vi "AddNormalPulseVoltammetry.vi"(0 "deviceName":string, 1 "channel":u8, 2 "repeats":u16=1, 3 "quietTime":sgl, 4 "quietTimeSamplingInterval":sgl=1.0, 5 "startVoltage":sgl, 6 "isStartVoltageVsOCP":bool, 7 "error in (no error)":errorcluster, 8 "endVoltage":sgl, 9 "isEndVoltageVsOCP":bool, 10 "vStep":sgl, 11 "pulseWidth":sgl, 12 "pulsePeriod":sgl, 13 "approxMaxCurrent":sgl=inf, 14 "isAutoRange":bool=TRUE, 15 "alphaFactor":sgl=75.0) -> (27 "error out":errorcluster)   [LabVIEW 2018]
doc: "EXPORT void AisAddNormalPulseVoltammetry(const char* deviceName, uint8_t channel, uint16_t repeats, float quietTime, float quietTimeSamplingInterval, float startVoltage, bool isStartVoltageVsOCP, float endVoltage, bool isEndVoltageVsOCP, float vStep, float pulseWidth, float pulsePeriod, float approxMaxCurrent, bool isAutoRange, float alphaFactor);"
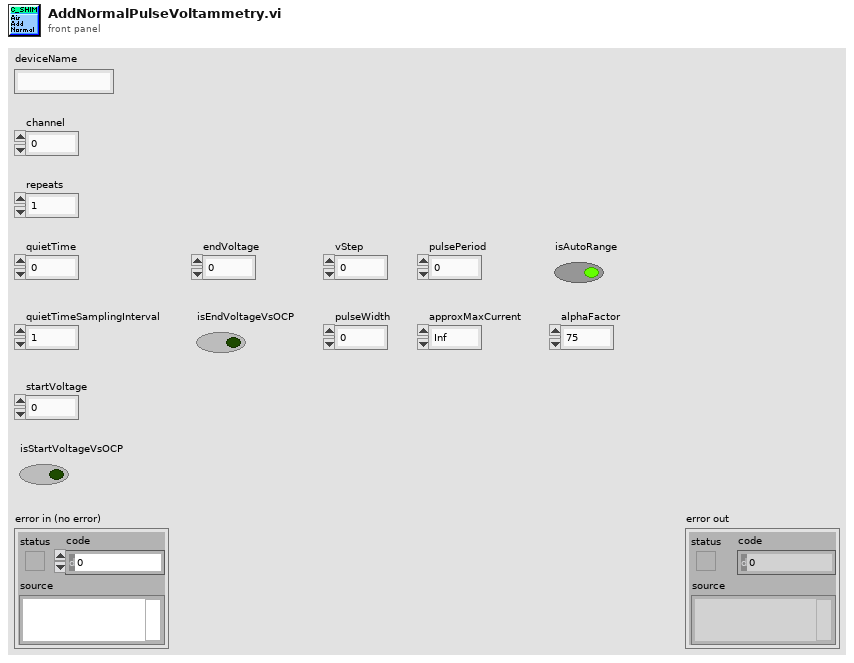
[diagram p1: front panel]
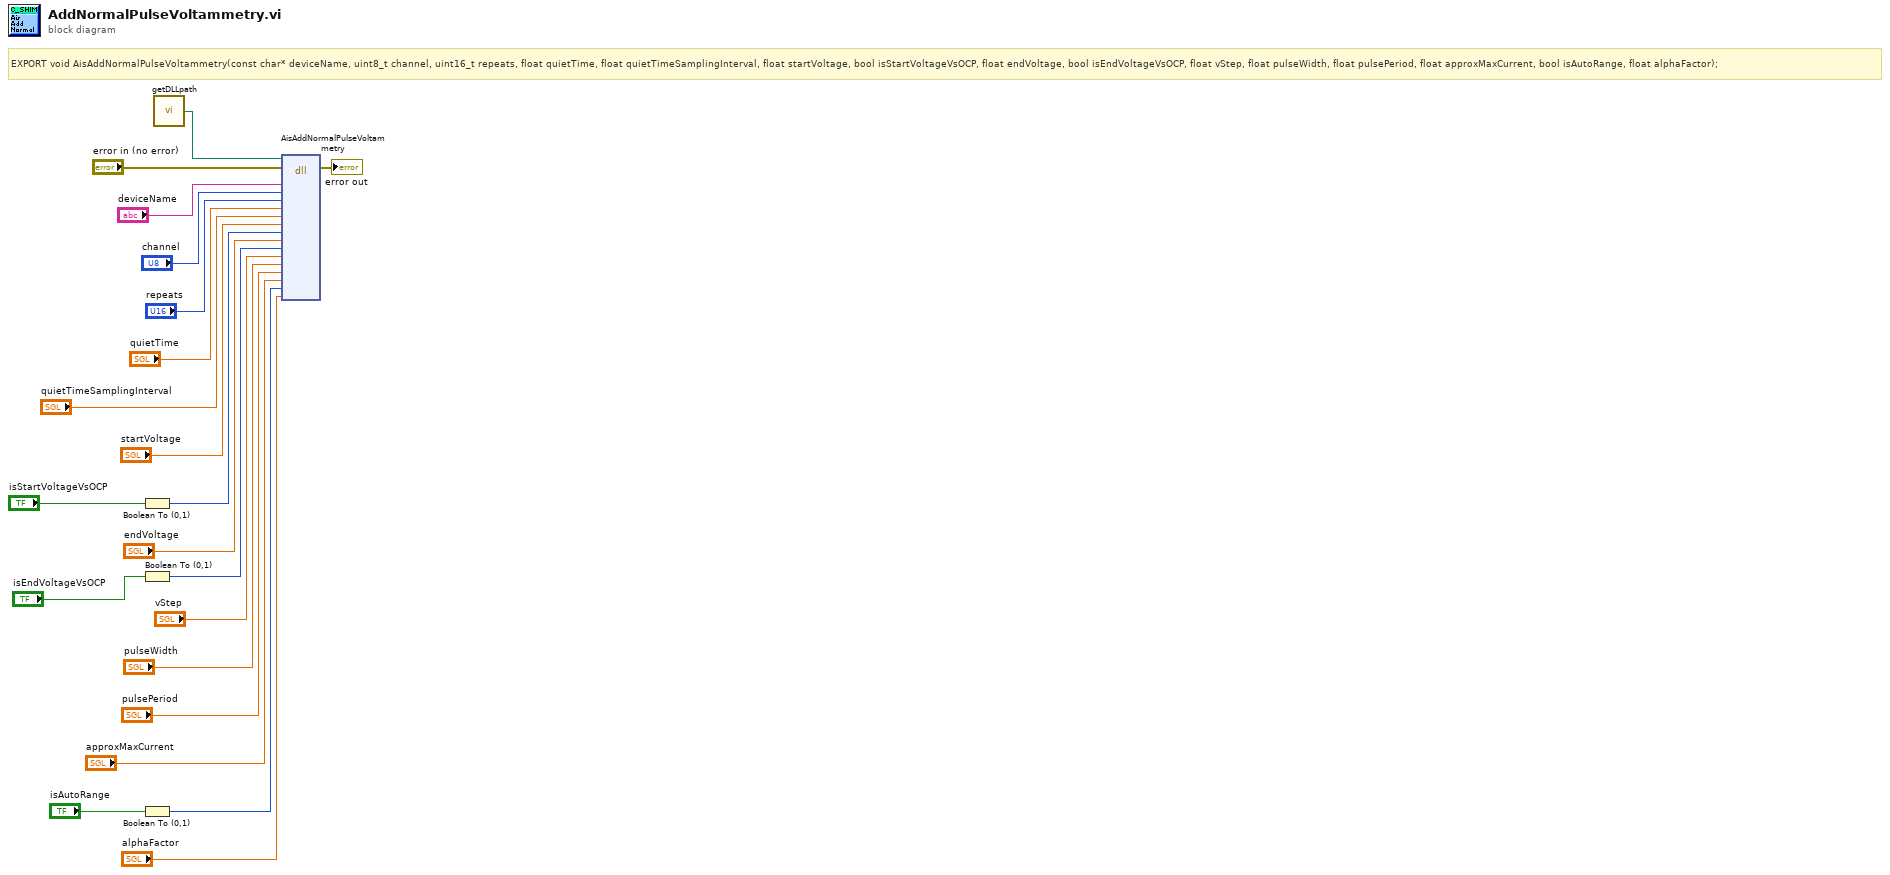
[diagram p0: block diagram]
diagram:
  # "EXPORT void AisAddNormalPulseVoltammetry(const char* deviceName, uint8_t channel, uint16_t repeats, float quietTime, float quietTimeSamplingInterval, float startVoltage, bool isStartVoltageVsOCP, float endVoltage, bool isEndVoltageVsOCP, float vStep, float pulseWidth, float pulsePeriod, float approxMaxCurrent, bool isAutoRange, float alphaFactor);"
  n1 = Boolean To (0,1)(Boolean="isStartVoltageVsOCP") -> (0, 1=w14:i16)
  n2 = Boolean To (0,1)(Boolean="isEndVoltageVsOCP") -> (0, 1=w11:i16)
  n3 = Boolean To (0,1)(Boolean="isAutoRange") -> (0, 1=w5:i16)
  n4 = call "getDLLpath.vi"() -> ("DLL_Path"=w1:path)
  n5 = dll-call lib="?" fn="AisAddNormalPulseVoltammetry"(path in=w1, error in="error in (no error)", "deviceName"="deviceName", "channel"="channel", "repeats"="repeats", "quietTime"="quietTime", "quietTimeSamplingInterval"="quietTimeSamplingInterval", "startVoltage"="startVoltage", "isStartVoltageVsOCP"=w14, "endVoltage"="endVoltage", "isEndVoltageVsOCP"=w11, "vStep"="vStep", "pulseWidth"="pulseWidth", "pulsePeriod"="pulsePeriod", "approxMaxCurrent"="approxMaxCurrent", "isAutoRange"=w5, "alphaFactor"="alphaFactor") -> (error out=→"error out":errorcluster)  [unwired: 17 in, 1 out]
